vi "Sourcetree difftool string.vi"() -> (3 "Sourcetree Difftool String":string="difftool \"sourcetree\"")   [LabVIEW 2016]
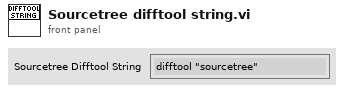
[diagram p1: front panel]
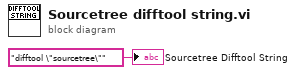
[diagram p0: block diagram]
diagram:
  "Sourcetree Difftool String" <- "difftool \"sourcetree\""
